vi "Launch Method.vi"(8 "error in (no error)":errorcluster, 9 "methodCall":T1, 10 "methodCall queue":refnum<queue>, 11 "vi path":path) -> (0 "error out":errorcluster)   [LabVIEW 2014]
uses:
  Controls/methodCall.ctl
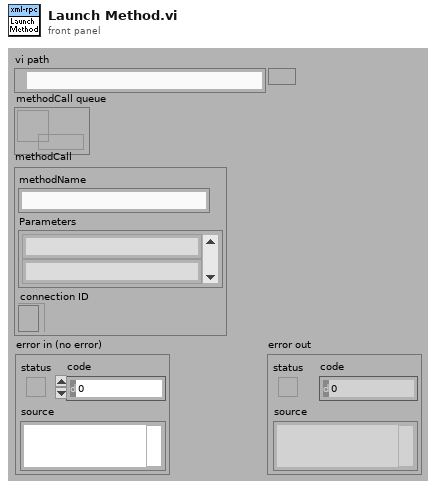
[diagram p1: front panel]
types:
  T1 = typedef "methodCall.ctl" = cluster{"methodName":string, "Parameters":string[], "connection ID":refnum<k5>}
  T2 = enum32{"Bad", "Idle", "Run top level", "Running"}
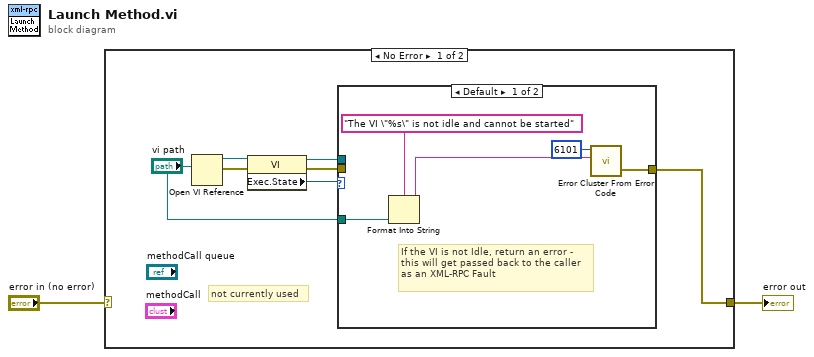
[diagram p0: block diagram]
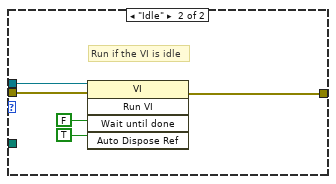
[diagram p2: hidden frame]
diagram:
  n1 = case shown="No Error" "error in (no error)" {
    selector: "error in (no error)" -> [_ w20]
    tunnel: [w4 w20] -> w1
    frame No Error {
      # "not currently used"
      n2 = Open VI Reference(vi path="vi path") -> (vi reference=w9:refnum<vi>, error out=w8:errorcluster)  [unwired: 5 in]
      n3 = property class="VI"(reference=w9, error in=w8) -> (reference out=w6:refnum<vi>, error out=w7:errorcluster, "Exec.State"=w5:T2)
      n4 = case shown="Default" w5 {
        tunnel: w7 -> [_ w17]
        tunnel: w6 -> [_ w16]
        tunnel: [w14 w15] -> w4
        tunnel: "vi path" -> [w13 _]
        frame Default {
          # "If the VI is not Idle, return an error - this will get passed back to the caller as an XML-RPC Fault"
          n5 = Format Into String(format string="The VI \"%s\" is not idle and cannot be started", w13) -> (resulting string=w11:string)  [unwired: 2 in, 1 out]
          n6 = call <vilib>:"Error Cluster From Error Code.vi"("error message (\"\")"=w11, "error code (0)"=6101) -> ("error out"=w14:errorcluster)  [unwired: 7 in]
        }
        frame "Idle" {
          # "Run if the VI is idle"
          n7 = invoke class="VI" method="Run VI"(reference=w16, error in=w17, "Wait until done"=FALSE ("Wait Until Done"), "Auto Dispose Ref"=TRUE ("Auto Dispose Reference")) -> (error out=w15:errorcluster)  [unwired: 1 in, 4 out]
        }
      }
    }
    frame Error {
    }
  }
  "error out" <- w1
